vi "Set Test Finder.vi"(8 "error in (no error)":errorcluster, 10 "Test Cases Found Registration":refnum<event-registration>, 11 "Icon Decorator In":refnum<class "Icon Decorator.lvclass">) -> (0 "error out":errorcluster, 3 "Icon Decorator Out":refnum<class "Icon Decorator.lvclass">)   [LabVIEW 2020, in "Icon Decorator.lvclass"]
uses:
  Icon Decorator.lvclass
  C:/Git/astemes-lunit/source/Application Framework/Process Classes/Process/Process.lvclass
  Application Framework/Process Classes/Process/Process.lvclass/Process.ctl
  Icon Decorator.lvclass/Icon Decorator.ctl
  Application Framework/Process Classes/Process/Process.lvclass
  C:/Git/astemes-lunit/source/Framework/Icon Decorator/Icon Decorator.lvclass
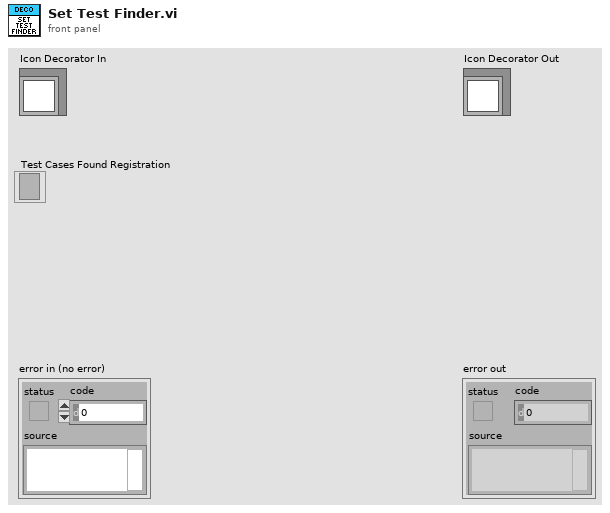
[diagram p1: front panel]
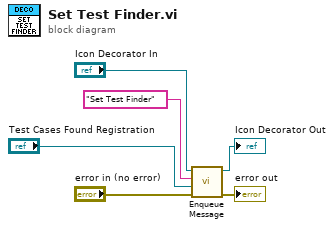
[diagram p0: block diagram]
diagram:
  n1 = call "Enqueue Message.vi"("error in (no error)"="error in (no error)", "Message Data"="Test Cases Found Registration", "Message"="Set Test Finder", "Process In"="Icon Decorator In") -> ("error out"=→"error out":errorcluster, "Process Out"=→"Icon Decorator Out":refnum<class "Icon Decorator.lvclass">)  [unwired: 6 in]
